vi "VXM-MoveRelative.vi"(8 "error in (no error)":errorcluster, 9 "Moves":T2[](array[typedef]), 11 "Message que":T1) -> (0 "error out":errorcluster)   [LabVIEW 2017]
uses:
  singleAxisMoveDef.ctl
  mmWaveAxis.ctl
  Support/MessageQue/MessageQue.ctl
  Support/MessageQue/MessageCluster.ctl
  Support/MessageQue/MessageQue.lvlib
panel:
  # "#TBD JUST ONE AXIS SUPPORTED NOW"
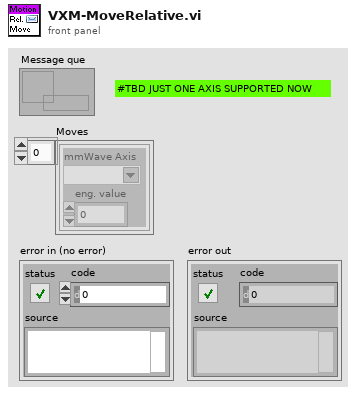
[diagram p1: front panel]
types:
  T1 = typedef "MessageQue.lvlib/MessageQue.ctl" = refnum<queue>
  T2 = typedef "singleAxisMoveDef.ctl" = cluster{"mmWave Axis":T3, "eng. value":dbl}
  T3 = typedef "mmWaveAxis.ctl" = string
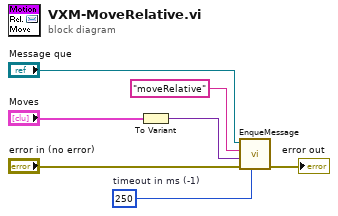
[diagram p0: block diagram]
diagram:
  w6 = 250  # timeout in ms (-1)
  n1 = To Variant(anything="Moves") -> (Variant=w7:variant)
  n2 = call "EnqueMessage.vi"("timeout in ms (-1)"=w6, "error in"="error in (no error)", "Message Payload"=w7, "Message Command"="moveRelative", "Message que"="Message que") -> ("error out"=→"error out":errorcluster)  [unwired: 5 in, 1 out]
